vi "Close.vi"(8 "error in":errorcluster, 11 "object in":refnum<class "Fgen VISA CFG.lvclass">) -> (0 "error out":errorcluster, 3 "object out":refnum<class "Fgen VISA CFG.lvclass">)   [LabVIEW 2023, in "Fgen VISA CFG.lvclass"]
uses:
  Fgen VISA CFG.lvclass
  Fgen VISA CFG.lvclass/Fgen VISA CFG.ctl
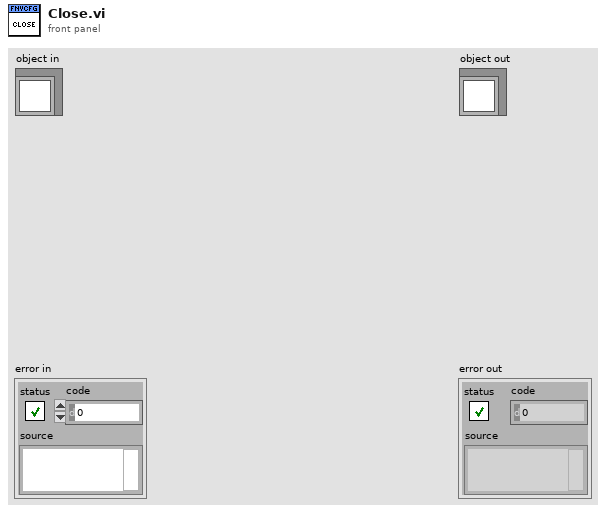
[diagram p1: front panel]
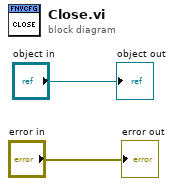
[diagram p0: block diagram]
diagram:
  "error out" <- "error in"
  "object out" <- "object in"
